vi "FGV_DevHandle.vi"(7 "Set":bool, 8 "error in (no error)":errorcluster caption="错误输入（无错误）", 9 "Name":string, 10 "Type":enum16{"Device", "Ch0", "Ch1"}(ring), 11 "handle":u64) -> (0 "error out":errorcluster caption="错误输出", 1 "Name out":string, 3 "handle out":u64)   [LabVIEW 2018, in "CAN FD.lvlib"]
uses:
  CAN FD.lvlib
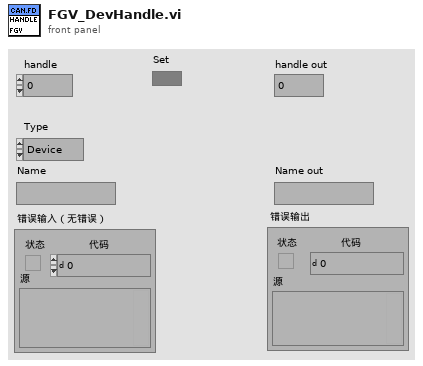
[diagram p1: front panel]
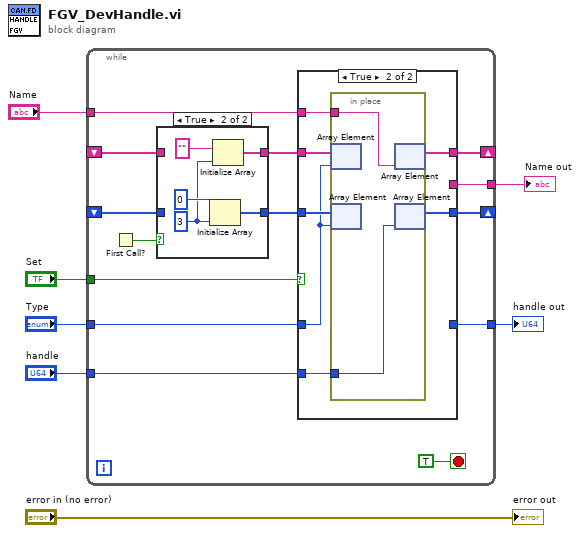
[diagram p0: block diagram]
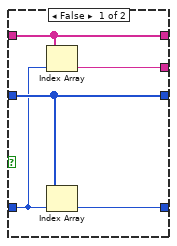
[diagram p2: hidden frame]
diagram:
  n1 = while {
    shift-right: [w17] -> _
    shift-left: _ -> [w19]
    tunnel: "Set" -> [w18]
    tunnel: "Type" -> [w15]
    tunnel: "handle" -> [w14]
    tunnel: [w13] -> w3
    shift-right: [w10] -> _
    shift-left: _ -> [w12]
    tunnel: "Name" -> [w9]
    tunnel: [w8] -> w1
    stop <- TRUE stop-if-true
    n2 = First Call?() -> (First Call?: T/F=w20:bool)
    n3 = case shown="True" w20 {
      tunnel: [w37 w41] -> w16
      tunnel: w19 -> [w37 _]
      tunnel: w12 -> [w36 _]
      tunnel: [w36 w40] -> w11
      frame False {
      }
      frame True {
        w39 = 3 ("维数大小")
        n4 = Initialize Array(u64 0 ("元素"), w39) -> (w41:u64[])
        n5 = Initialize Array("", w39) -> (w40:string[])
      }
    }
    n6 = case shown="True" w18 {
      tunnel: [w26 w32] -> w17
      tunnel: w16 -> [w26 w33]
      tunnel: w15 -> [w23 w28]
      tunnel: w14 -> [_ w31]
      tunnel: [w25 _] -> w13
      tunnel: w11 -> [w24 w30]
      tunnel: [w24 w29] -> w10
      tunnel: w9 -> [_ w27]
      tunnel: [w22 _] -> w8
      frame False {
        n7 = Index Array(array=w24, index=w23) -> (element=w22:string)
        n8 = Index Array(array=w26, index=w23) -> (element=w25:u64)
      }
      frame True {
        n9 = in-place {
          in-place-border: w31 -> [w35]
          in-place-border: w27 -> [w34]
          n10 = in-place-array #1(w30, w28) -> ()  [unwired: 1 out]
          n11 = in-place-array #2(w33, w28) -> ()  [unwired: 1 out]
          n12 = in-place-array #1(w34) -> (w29:string[])  [unwired: 1 out]
          n13 = in-place-array #2(w35) -> (w32:u64[])  [unwired: 1 out]
        }
      }
    }
  }
  "handle out" <- w3
  "Name out" <- w1
  "error out" <- "error in (no error)"
